vi "Disabled Property(Main Controls)_Initialize.vi"(8 "error in (no error)":errorcluster, 11 "MWWL Verification in":refnum<class "MWWL Verification.lvclass">) -> (0 "error out":errorcluster, 3 "MWWL Verification out":refnum<class "MWWL Verification.lvclass">)   [LabVIEW 2018, in "MWWL Verification.lvlib" / "MWWL Verification.lvclass"]
uses:
  MWWL Verification.lvclass
  MWWL Verification.lvclass/MWWL Verification.ctl
types:
  T1 = enum8{"Enabled", "Disabled", "Disabled and Grayed Out"}
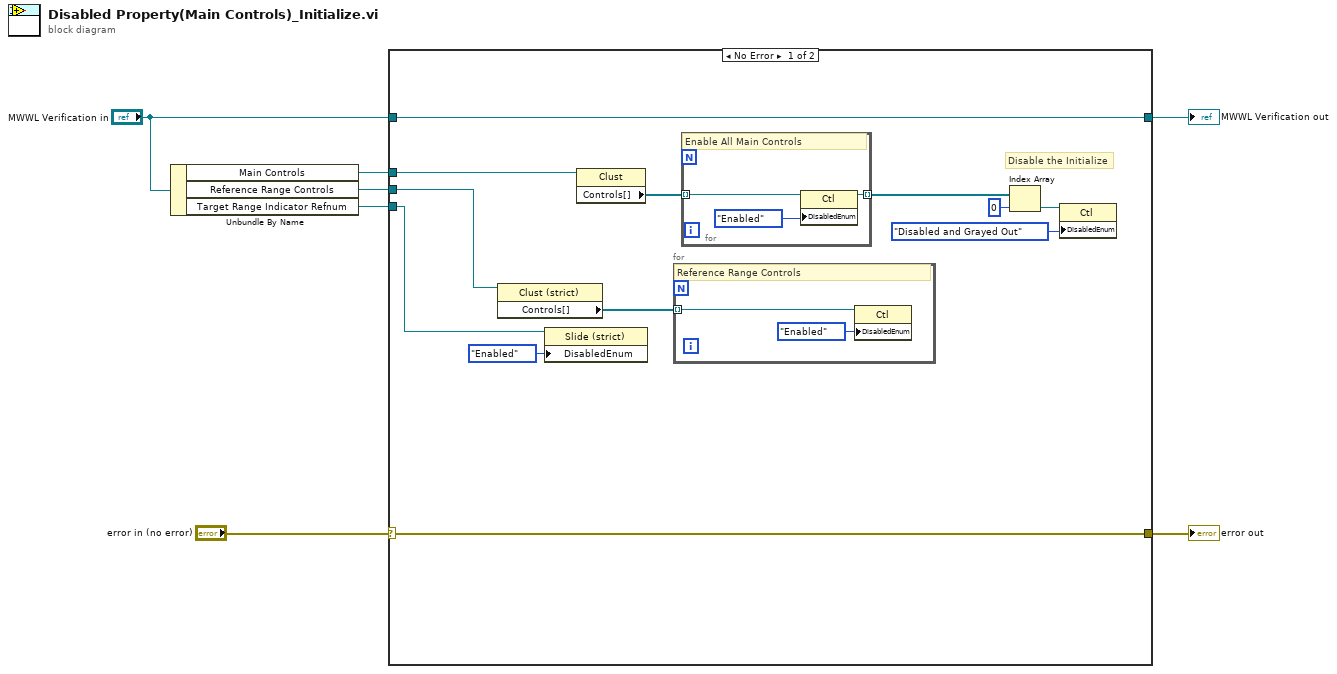
[diagram p0: block diagram]
diagram:
  n1 = Unbundle By Name("MWWL Verification in") -> ("Main Controls"=w3:refnum<vi>, "Reference Range Controls"=w2:refnum<vi>, "Target Range Indicator Refnum"=w1:refnum<vi>)
  n2 = case shown="No Error" "error in (no error)" {
    selector: "error in (no error)" -> [w18 w26]
    tunnel: [w18 w26] -> w6
    tunnel: [w19 w25] -> w5
    tunnel: "MWWL Verification in" -> [w19 w25]
    tunnel: w3 -> [w17 _]
    tunnel: w2 -> [w16 _]
    tunnel: w1 -> [w9 _]
    frame No Error {
      # "Disable the Initialize"
      n3 = property class="Clust (strict)"(reference=w16) -> ("Controls[]"=w15:refnum<vi>[])  [unwired: 1 in, 2 out]
      n4 = property class="Slide (strict)"(reference=w9, "DisabledEnum"=T1."Enabled" ("Disabled")) -> ()  [unwired: 1 in, 2 out]
      n5 = property class="Clust"(reference=w17) -> ("Controls[]"=w14:refnum<vi>[])  [unwired: 1 in, 2 out]
      n6 = for {
        tunnel: w15 -> [w23] mode=indexing
        # "Reference Range Controls"
        n7 = property class="Ctl"(reference=w23, "DisabledEnum"=T1."Enabled" ("Disabled")) -> ()  [unwired: 1 in, 2 out]
      }
      n8 = for {
        tunnel: w14 -> [w21] mode=indexing
        tunnel: [w20] -> w8 mode=indexing
        # "Enable All Main Controls"
        n9 = property class="Ctl"(reference=w21, "DisabledEnum"=T1."Enabled" ("Disabled")) -> (reference out=w20:refnum<vi>)  [unwired: 1 in, 1 out]
      }
      n10 = Index Array(array=w8, index=0) -> (element=w11:refnum<vi>)
      n11 = property class="Ctl"(reference=w11, "DisabledEnum"=T1."Disabled and Grayed Out" ("Disabled")) -> ()  [unwired: 1 in, 2 out]
    }
    frame Error {
    }
  }
  "error out" <- w6
  "MWWL Verification out" <- w5
